vi "Remove Panel.vi"(8 "error in (no error)":errorcluster, 10 "Panel":string) -> (0 "error out":errorcluster)   [LabVIEW 2017, in "MGI-Panel Manager.lvlib" / "Panel Registry.lvclass"]
doc: "Removes a panel.\n\n----\nPlease see the following web address for additional documentation and tutorial information:\nhttp://www.mooregoodideas.com/mgi-panel-manager/\n\nAuthor: Derek Trepanier\n\nCopyright (c) 2018, Moore Good Ideas, Inc.\n\nAll rights reserved.\n\nRedistribution and use in source and binary forms, with or without modification, are permitted provided that the following conditions are met:\n\n * Redistributions of source code must retain the above copyright notice, this list of conditions and the following disclaimer.\n * Redistributions in binary form must reproduce the above copyright notice, this list of conditions and the following disclaimer in the documentation and/or other materials provided with the distribution.\n * Neither the name of Moore Good Ideas, Inc. nor the names of its contributors may be used to endorse or promote products derived from this software without specific prior written permission.\n\nTHIS SOFTWARE IS PROVIDED BY THE COPYRIGHT HOLDERS AND CONTRIBUTORS \"AS IS\" AND ANY EXPRESS OR IMPLIED WARRANTIES, INCLUDING, BUT NOT LIMITED TO, THE IMPLIED WARRANTIES OF MERCHANTABILITY AND FITNESS FOR A PARTICULAR PURPOSE ARE DISCLAIMED. IN NO EVENT SHALL THE COPYRIGHT OWNER OR CONTRIBUTORS BE LIABLE FOR ANY DIRECT, INDIRECT, INCIDENTAL, SPECIAL, EXEMPLARY, OR CONSEQUENTIAL DAMAGES (INCLUDING, BUT NOT LIMITED TO, PROCUREMENT OF SUBSTITUTE GOODS OR SERVICES; LOSS OF USE, DATA, OR PROFITS; OR BUSINESS INTERRUPTION) HOWEVER CAUSED AND ON ANY THEORY OF LIABILITY, WHETHER IN CONTRACT, STRICT LIABILITY, OR TORT (INCLUDING NEGLIGENCE OR OTHERWISE) ARISING IN ANY WAY OUT OF THE USE OF THIS SOFTWARE, EVEN IF ADVISED OF THE POSSIBILITY OF SUCH DAMAGE."
uses:
  Panel Registry.lvclass
  Cursor/Cursor.lvclass
  Cursor/Lookup Actions.ctl
  Panel Helper/Events.ctl
  Panel Helper/Panel Helper.lvclass
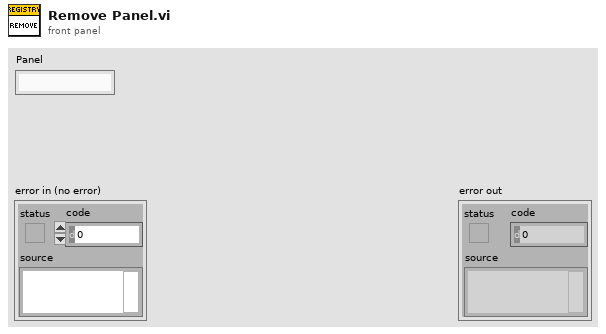
[diagram p1: front panel]
types:
  T1 = typedef "MGI-Panel Manager.lvlib/Cursor.lvclass/Lookup Actions.ctl" = enum16{"Init", "Get", "Destroy"}
  T2 = typedef "MGI-Panel Manager.lvlib/Panel Helper.lvclass/Events.ctl" = enum16{"Initialized", "Shown", "Hidden", "Closed"}
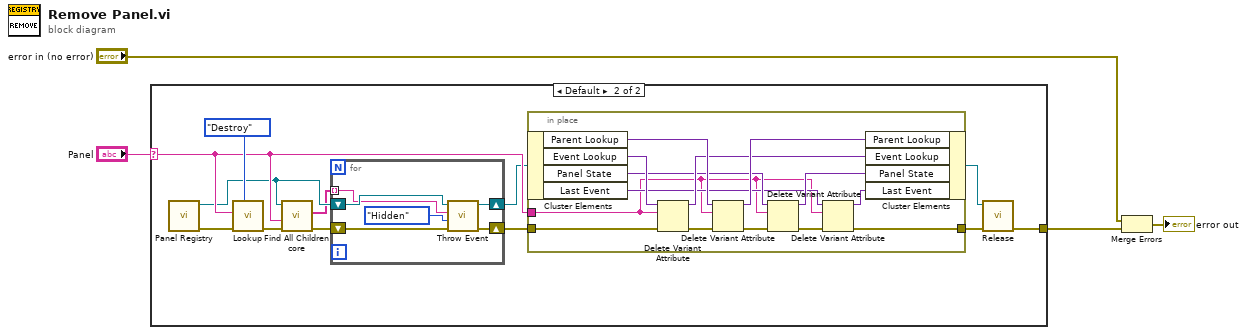
[diagram p0: block diagram]
diagram:
  n1 = case shown="Default" "Panel" {
    selector: "Panel" -> [_ w11]
    tunnel: [_ w16] -> w4
    frame "" {
    }
    frame Default {
      n2 = call "Panel Registry.vi"() -> ("error out"=w12:errorcluster, "Panel Registry out"=w9:refnum<class "Panel Registry.lvclass">)  [unwired: 10 in]
      n3 = call "Lookup.vi"("Action"=Lookup_Actions."Destroy", "error in (no error)"=w12, "Top Level VI"=w11) -> ("error out"=w10:errorcluster)  [unwired: 7 in, 1 out]
      n4 = call "Find All Children core.vi"("error in (no error)"=w10, "Panel"=w11, "Panel Registry in"=w9) -> ("error out"=w7:errorcluster, "All Children"=w5:string[])  [unwired: 7 in]
      n5 = for {
        shift-right: [w21] -> w8
        shift-left: w9 -> [w22]
        shift-right: [w19] -> w6
        shift-left: w7 -> [w20]
        tunnel: w5 -> [w17] mode=indexing
        n6 = call "Throw Event.vi"("error in (no error)"=w20, "Event"=Events."Hidden", "Panel"=w17, "Panel Registry in"=w22) -> ("error out"=w19:errorcluster, "Panel Registry out"=w21:refnum<class "Panel Registry.lvclass">)  [unwired: 6 in]
      }
      n7 = in-place {
        in-place-border: w11 -> [w25]
        in-place-border: [w23] -> w14
        in-place-border: w6 -> [w32]
        n8 = in-place-cluster #1(w8) -> ("Parent Lookup"=w36:variant, "Event Lookup"=w29:variant, "Panel State"=w28:variant, "Last Event"=w27:variant)
        n9 = Delete Variant Attribute(4:w32, 6:w25, 7:w29) -> (0:w33:errorcluster, 3:w34:variant)  [unwired: 1 out]
        n10 = Delete Variant Attribute(4:w33, 6:w25, 7:w36) -> (0:w30:errorcluster, 3:w35:variant)  [unwired: 1 out]
        n11 = Delete Variant Attribute(4:w30, 6:w25, 7:w28) -> (0:w24:errorcluster, 3:w31:variant)  [unwired: 1 out]
        n12 = Delete Variant Attribute(4:w24, 6:w25, 7:w27) -> (0:w23:errorcluster, 3:w26:variant)  [unwired: 1 out]
        n13 = in-place-cluster #1("Parent Lookup"=w35, "Event Lookup"=w34, "Panel State"=w31, "Last Event"=w26) -> (w15:refnum<class "Panel Registry.lvclass">)
      }
      n14 = call "Release.vi"("error in (no error)"=w14, "Panel Registry in"=w15) -> ("error out"=w16:errorcluster)  [unwired: 9 in]
    }
  }
  n15 = Merge Errors("error in (no error)", w4) -> (→"error out":errorcluster)
